vi "voltage_variation.vi"(8 "t_end":dbl[](array[numeric]), 9 "t_start":dbl[](array[numeric]), 10 "v_rms":dbl[](array[numeric])) -> (1 "pre_V_rms":dbl[](array[numeric]), 2 "V_variation":dbl[](array[numeric]))   [LabVIEW 2014]
uses:
  <vilib>/imath/engines/lvmath2/RunTimeEngine/BuiltInFunctions/is_empty/NIMS_is_empty(GV).vi
  <instcachedir>/0/NIMS_is_empty(GV)_FC7E7C3D9544432CB6AA2416ADCF6D56.lvgen/NIMS_is_empty(GV)_FC7E7C3D9544432CB6AA2416ADCF6D56_001.vi
  <vilib>/imath/engines/lvmath2/RunTimeEngine/BuiltInFunctions/length/NIMS_length(GV).vi
  <instcachedir>/0/NIMS_length(GV)_08A3D13377FD4E4B96F5795FBF3698FA.lvgen/NIMS_length(GV)_08A3D13377FD4E4B96F5795FBF3698FA_000.vi
  <vilib>/imath/engines/lvmath2/RunTimeEngine/BuiltInFunctions/zeros/NIMS_V=zeros(I32,I32).vi
  <vilib>/imathl/engines/lvmath/Functions/Error Handling/Create Error.vi
  <vilib>/imath/engines/lvmath2/RunTimeEngine/RangeToken/NIMS_Range_R2 - Integer.vi
  <instcachedir>/0/NIMS_Range_R2 - Integer_2D1304BAF97744E0A293025746CBADFC.lvgen/NIMS_Range_R2 - Integer_2D1304BAF97744E0A293025746CBADFC_000.vi
  <vilib>/imath/engines/lvmath2/RunTimeEngine/CommandStatement/MC_CommandStatement_break.vi
  <vilib>/imath/engines/lvmath2/RunTimeEngine/IndexRead/NIMS V(S).vi
  <instcachedir>/0/NIMS V(S)_0488751826AF41519A22953C041130DC.lvgen/NIMS V(S)_0488751826AF41519A22953C041130DC_000.vi
  <vilib>/imath/engines/lvmath2/RunTimeEngine/RangeToken/NIMS_Range.vi
  <instcachedir>/0/NIMS_Range_9BCE657718DF4976A877346C61F22738.lvgen/NIMS_Range_9BCE657718DF4976A877346C61F22738_000.vi
  <vilib>/imath/engines/lvmath2/RunTimeSupport/NIMS_Error if Not Equal.vi
  <instcachedir>/0/NIMS_Error if Not Equal_8A0E9F659B9142D69417CC259581C4FD.lvgen/NIMS_Error if Not Equal_8A0E9F659B9142D69417CC259581C4FD_001.vi
  <vilib>/imath/engines/lvmath2/RunTimeEngine/IndexRead/NIMS M(S,V).vi
  <instcachedir>/0/NIMS M(S,V)_5C1965D37F59432CA0E9661793EAFE90.lvgen/NIMS M(S,V)_5C1965D37F59432CA0E9661793EAFE90_000.vi
  <vilib>/imath/engines/lvmath2/RunTimeEngine/BuiltInFunctions/mean/NIMS_RS=mean(RV,I32).vi
  <vilib>/imath/engines/lvmath2/RunTimeEngine/IndexReplace/NIMS V(S)=S.vi
  <instcachedir>/0/NIMS V(S)=S_2D52C4EC15D8415E870AEE69FB516CCA.lvgen/NIMS V(S)=S_2D52C4EC15D8415E870AEE69FB516CCA_000.vi
  <vilib>/imath/engines/lvmath2/RunTimeEngine/ErrorHandling/NIMS_Create Error From Enums.vi
  <vilib>/imath/engines/lvmath2/RunTimeEngine/BuiltInFunctions/min/1 input/NIMS_min(RV).vi
  <instcachedir>/0/NIMS_min(RV)_EE2DD3E2888846108C5160A664B67832.lvgen/NIMS_min(RV)_EE2DD3E2888846108C5160A664B67832_000.vi
  <vilib>/imath/engines/lvmath2/RunTimeEngine/BuiltInFunctions/max/1 input/NIMS_max(RV).vi
  <instcachedir>/0/NIMS_max(RV)_237633DB1D604D5BA7001287DF3C7957.lvgen/NIMS_max(RV)_237633DB1D604D5BA7001287DF3C7957_000.vi
  <vilib>/imath/engines/lvmath2/RunTimeEngine/BuiltInFunctions/abs/NIMS_abs(signed).vi
  <instcachedir>/0/NIMS_abs(signed)_C4FCB8E6058B49B797C7C8D53CA5F6EC.lvgen/NIMS_abs(signed)_C4FCB8E6058B49B797C7C8D53CA5F6EC_000.vi
  <vilib>/imath/engines/lvmath2/RunTimeEngine/NodeEndStatement/NIMS_NodeEndStatement_Output.vi
  <instcachedir>/0/NIMS_NodeEndStatement_Output_53EC0D466D134D7ABD903AC30B43404B.lvgen/NIMS_NodeEndStatement_Output_53EC0D466D134D7ABD903AC30B43404B_005.vi
  <vilib>/imath/engines/lvmath2/RunTimeEngine/ErrorHandling/NIMS_Finalize Error.vi
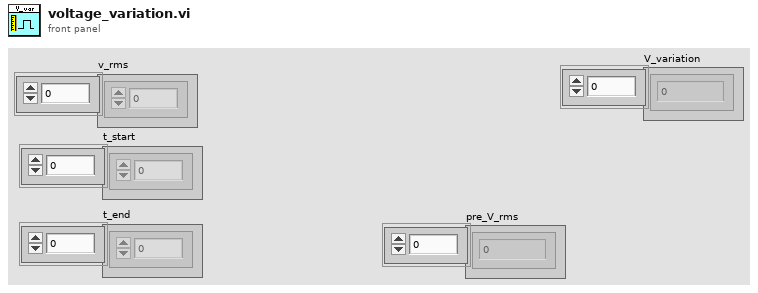
[diagram p1: front panel]
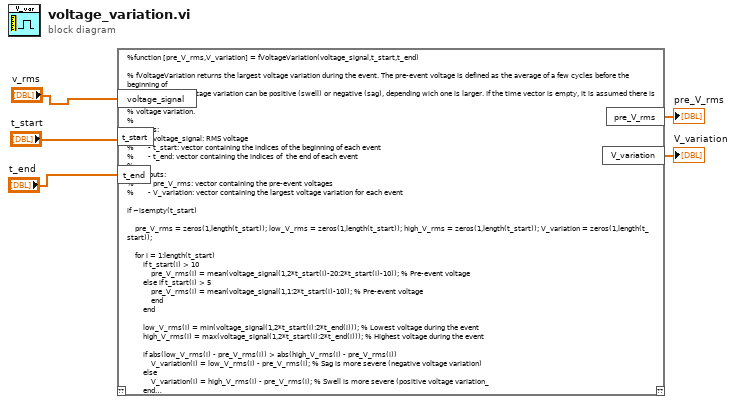
[diagram p0: block diagram]
diagram:
  n1 = mathscript code="%function [pre_V_rms,V_variation] = fVoltageVariation(voltage_signal,t_start,t_end)\n\n% fVoltageVariation returns the largest voltage variation during the event. The pre-event voltage is defined as the average of a few cycles before the beginning of\n% the event. The voltage variation can be positive (swell) or negative (sag), depending wich one is larger. If the time vector is empty, it is assumed there is no\n% voltage variation.\n%\n% Inputs:\n%       - voltage_signal: RMS voltage\n%       - t_start: vector containing the indices of the beginning of each event\n%       - t_end: vector containing the indices of  the end of each event\n%\n% Outputs:\n%       - pre_V_rms: vector containing the pre-event voltages\n%       - V_variation: vector containing the largest voltage variation for each event\n\nif ~isempty(t_start)\n    \n    pre_V_rms = zeros(1,length(t_start)); low_V_rms = zeros(1,length(t_start)); high_V_rms = zeros(1,length(t_start)); V_variation = zeros(1,length(t_start));    \n    \n    for i = 1:length(t_start)\n        if t_start(i) > 10\n            pre_V_rms(i) = mean(voltage_signal(1,2*t_start(i)-20:2*t_start(i)-10)); % Pre-event voltage\n        else if t_start(i) > 5\n            pre_V_rms(i) = mean(voltage_signal(1,1:2*t_start(i)-10)); % Pre-event voltage\n            end\n        end\n\n        low_V_rms(i) = min(voltage_signal(1,2*t_start(i):2*t_end(i))); % Lowest voltage during the event\n        high_V_rms(i) = max(voltage_signal(1,2*t_start(i):2*t_end(i))); % Highest voltage during the event\n        \n        if abs(low_V_rms(i) - pre_V_rms(i)) > abs(high_V_rms(i) - pre_V_rms(i))\n            V_variation(i) = low_V_rms(i) - pre_V_rms(i); % Sag is more severe (negative voltage variation)\n        else\n            V_variation(i) = high_V_rms(i) - pre_V_rms(i); % Swell is more severe (positive voltage variation_\n        end\n    end\nelse\n    pre_V_rms = 1; \n    V_variation = 0; % No voltage variation (no event)\nend"("voltage_signal"="v_rms", "t_start"="t_start", "t_end"="t_end") -> ("pre_V_rms"=→"pre_V_rms":dbl[], "V_variation"=→"V_variation":dbl[])  [unwired: 1 in, 1 out]
